vi "arduinoSerialCommunication.vi"(9 "arduino COM port":refnum<visa-resource-name>="Arduino", 11 "Array 2":bool[](array[boolean])) -> ()   [LabVIEW 2020]
uses:
  <vilib>/Instr/_visa.llb/VISA Configure Serial Port (Instr).vi
panel:
  out "String 2":string
  out "String":string
  out "error out":errorcluster
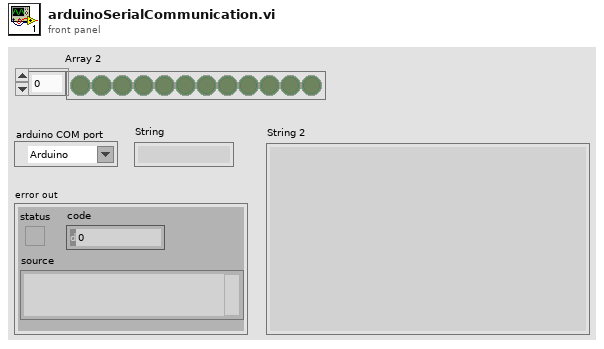
[diagram p1: front panel]
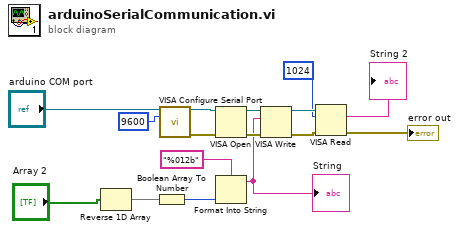
[diagram p0: block diagram]
diagram:
  n1 = Reverse 1D Array(array="Array 2") -> (reversed array=w2:bool[])
  n2 = Boolean Array To Number(Boolean array=w2) -> (number=w1:u32)
  n3 = call-poly "VISA Configure Serial Port"("VISA resource name"="arduino COM port", "baud rate (9600)"=9600) -> ("VISA resource name out"=w13:refnum<visa-resource-name>, "error out"=w12:errorcluster)  [unwired: 12 in]
  n4 = VISA Open(error in (no error)=w12, VISA resource name=w13) -> (VISA resource name=w11:refnum<visa-resource-name>, error out=w10:errorcluster)  [unwired: 3 in]
  n5 = Format Into String(format string="%012b", w1) -> (resulting string=w9:string)  [unwired: 2 in, 1 out]
  "String" <- w9
  n6 = VISA Write(VISA resource name=w11, write buffer=w9, error in (no error)=w10) -> (VISA resource name out=w8:refnum<visa-resource-name>, error out=w7:errorcluster)  [unwired: 1 out]
  n7 = VISA Read(VISA resource name=w8, byte count=1024, error in (no error)=w7) -> (read buffer=→"String 2":string, error out=→"error out":errorcluster)  [unwired: 2 out]
